vi "Configure Trigger.vi"(0 "VISA resource name":refnum<visa-resource-name>, 1 "Trigger Type (0: Continuous)":u16(ring) items=["Continuous", "Single", "Gate", "Segment Advance"], 2 "Trigger Source (0: Key)":u16(ring) items=["Key", "External", "Bus"], 5 "Modulation Format (0: Custom)":u16(ring) items=["Custom", "Dual Modulation", "Dual ARB"], 7 "Continuous Trigger Type (0: Free)":u16(ring) items=["Free", "Trigger", "Reset"], 9 "Retriggering Mode (0: ON)":u16(ring) items=["On", "Off", "Immediate"], 11 "error in (no error)":errorcluster, 12 "Gate Active (0: High)":u16(ring) items=["High", "Low"], 13 "Segment Advance Trigger Type (0: Continuous)":u16(ring) items=["Continuous", "Single"]) -> (4 "VISA resource name out":refnum<visa-resource-name>, 15 "error out":errorcluster)   [LabVIEW 2009, in "Agilent PSG MXG Series.lvlib"]
doc: "Configures the trigger source and trigger type for the specific modulation format.\n\n<B>Notes:</B>\n(1) This VI is valid only in E8267C, E8267D, N5182A.\n\n(2) For E8267C, this VI is valid only when the instrument installs <B>Option 002</B> (Internal baseband generator) or <B>Option 602</B> (Digital bus baseband generator).\n\n(3) For E8267D, this VI is valid only when the instrument installs <B>Option 601</B> or <B>Option 602</B> (Internal baseband generator).\n\n(4) For N5182A, this VI is valid only when the instrument installs <B>Option 651</B> or <B>Option 652</B> or <B>Option 654</B> (Internal baseband generator)."
uses:
  Agilent PSG MXG Series.lvlib
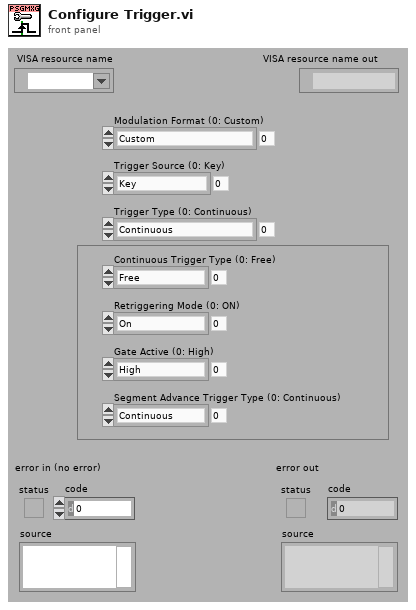
[diagram p1: front panel]
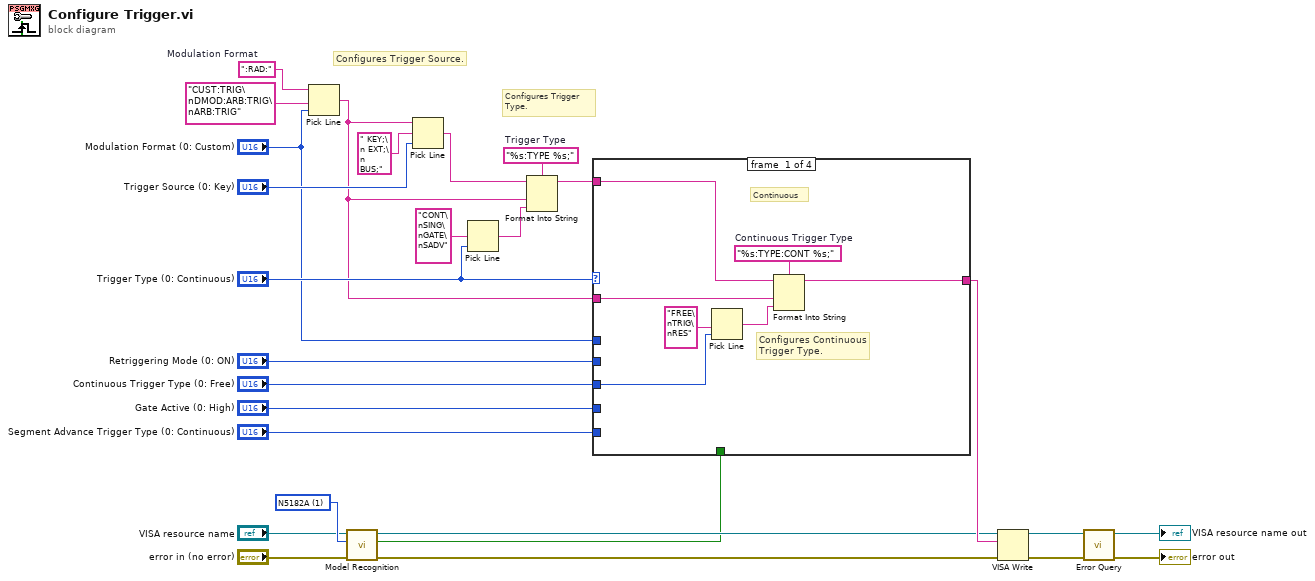
[diagram p0: block diagram]
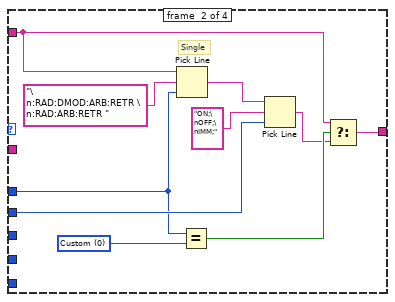
[diagram p2: hidden frame]
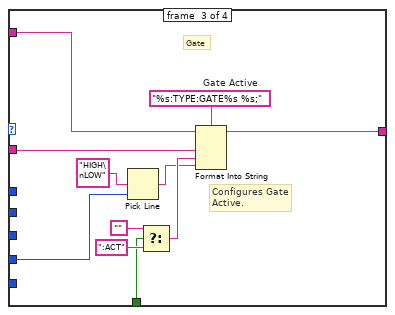
[diagram p3: hidden frame]
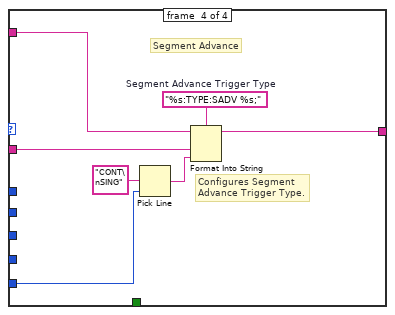
[diagram p4: hidden frame]
diagram:
  w11 = u16 1 items=["N5181A"=0, "N5182A"=1, "E8241A"=5, "E8244A"=6, "E8251A"=7, "E8254A"=8, "E8247C"=10, "E8257C"=11, "E8267C"=12, "E8257D"=15, "E8267D"=16] ("Model Type (0: N5181A)")
  w22 = "%s:TYPE %s;"  # Trigger Type
  w27 = ":RAD:"  # Modulation Format
  # "Configures Trigger\nType."
  # "Configures Trigger Source."
  n1 = Pick Line(string ("")=w27, multi-line string="CUST:TRIG\nDMOD:ARB:TRIG\nARB:TRIG", line index="Modulation Format (0: Custom)") -> (output string=w18:string)
  n2 = call "Model Recognition.vi"("error in (no error)"="error in (no error)", "Model Type (0: N5181A)"=w11, "VISA resource name"="VISA resource name") -> ("error out"=w9:errorcluster, "Is Model Correct"=w1:bool, "VISA resource name out"=w10:refnum<visa-resource-name>)  [unwired: 6 out]
  n3 = Pick Line(string ("")=w18, multi-line string=" KEY;\n EXT;\n BUS;" ("Trigger Source"), line index="Trigger Source (0: Key)") -> (output string=w23:string)
  n4 = Pick Line(multi-line string="CONT\nSING\nGATE\nSADV", line index="Trigger Type (0: Continuous)") -> (output string=w21:string)  [unwired: 1 out]
  n5 = Format Into String(format string=w22, initial string=w23, w18, w21) -> (resulting string=w17:string)  [unwired: 1 in, 1 out]
  n6 = case shown="0, Default" "Trigger Type (0: Continuous)" {
    tunnel: w18 -> [w33 _ w54 w61]
    tunnel: w17 -> [w30 w36 w51 w57]
    tunnel: "Continuous Trigger Type (0: Free)" -> [w29 _ _ _]
    tunnel: "Gate Active (0: High)" -> [_ _ w52 _]
    tunnel: "Segment Advance Trigger Type (0: Continuous)" -> [_ _ _ w58]
    tunnel: [w28 w35 w50 w56] -> w14
    tunnel: "Retriggering Mode (0: ON)" -> [_ w41 _ _]
    tunnel: "Modulation Format (0: Custom)" -> [_ w40 _ _]
    tunnel: w1 -> [_ _ w45 _]
    frame #0 {
      w34 = "%s:TYPE:CONT %s;"  # Continuous Trigger Type
      # "Configures Continuous\nTrigger Type."
      # "Continuous"
      n7 = Pick Line(multi-line string="FREE\nTRIG\nRES", line index=w29) -> (output string=w32:string)  [unwired: 1 out]
      n8 = Format Into String(format string=w34, initial string=w30, w33, w32) -> (resulting string=w28:string)  [unwired: 1 in, 1 out]
    }
    frame #1 {
      w39 = u16 0 items=["Custom", "Dual Modulation", "Dual ARB"] ("Format (0: Custom)")
      # "Single"
      n9 = Pick Line(string ("")=w36, multi-line string="\n:RAD:DMOD:ARB:RETR \n:RAD:ARB:RETR ", line index=w40) -> (output string=w43:string)
      n10 = Equal?(x=w40, y=w39) -> (x = y?=w38:bool)
      n11 = Pick Line(string ("")=w43, multi-line string="ON;\nOFF;\nIMM;", line index=w41) -> (output string=w37:string)
      n12 = Select(t=w36, s=w38, f=w37) -> (s? t:f=w35:string)
    }
    frame #2 {
      w55 = "%s:TYPE:GATE%s %s;"  # Gate Active
      # "Configures Gate\nActive."
      # "Gate"
      n13 = Pick Line(multi-line string="HIGH\nLOW", line index=w52) -> (output string=w48:string)  [unwired: 1 out]
      n14 = Select(t="", s=w45, f=":ACT") -> (s? t:f=w49:string)
      n15 = Format Into String(format string=w55, initial string=w51, w54, w49, w48) -> (resulting string=w50:string)  [unwired: 1 in, 1 out]
    }
    frame #3 {
      w62 = "%s:TYPE:SADV %s;"  # Segment Advance Trigger Type
      # "Configures Segment\nAdvance Trigger Type."
      # "Segment Advance"
      n16 = Pick Line(multi-line string="CONT\nSING", line index=w58) -> (output string=w60:string)  [unwired: 1 out]
      n17 = Format Into String(format string=w62, initial string=w57, w61, w60) -> (resulting string=w56:string)  [unwired: 1 in, 1 out]
    }
  }
  n18 = VISA Write(VISA resource name=w10, write buffer=w14, error in (no error)=w9) -> (VISA resource name out=w13:refnum<visa-resource-name>, error out=w12:errorcluster)  [unwired: 1 out]
  n19 = call "Error Query.vi"("error in (no error)"=w12, "VISA resource name"=w13) -> ("error out"=→"error out":errorcluster, "VISA resource name out"=→"VISA resource name out":refnum<visa-resource-name>)  [unwired: 8 out]
